vi "Get Package ID.vi"(0 "SystemLink repo in":T1, 7 "package name":string, 9 "package version":string, 11 "error in (no error)":errorcluster) -> (4 "SystemLink repo out":T1, 8 "package ID":string, 15 "error out":errorcluster)   [LabVIEW 2017, in "SystemLink_Repo_API.lvlib"]
doc: "Returns the Package ID for the specified Package Name and Package Version.\n\nError Handling:\nReturns an error if the specified package and version does not exist in the SystemLink repository."
uses:
  SystemLink_Repo_API.lvlib
  systemlink repo.ctl
  <vilib>/httpClient/ClientHandle.ctl
  <vilib>/httpClient/LabVIEWHTTPClient.lvlib
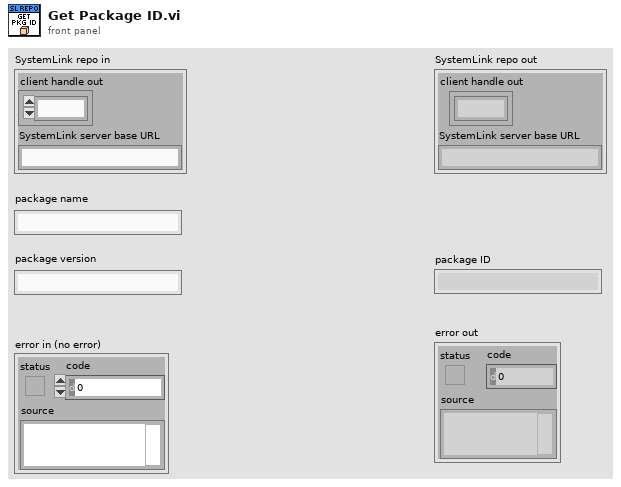
[diagram p1: front panel]
types:
  T1 = typedef "SystemLink_Repo_API.lvlib/systemlink repo.ctl" = cluster{"client handle out":T2, "SystemLink server base URL":string}
  T2 = typedef "LabVIEWHTTPClient.lvlib/ClientHandle.ctl" = refnum<k1>
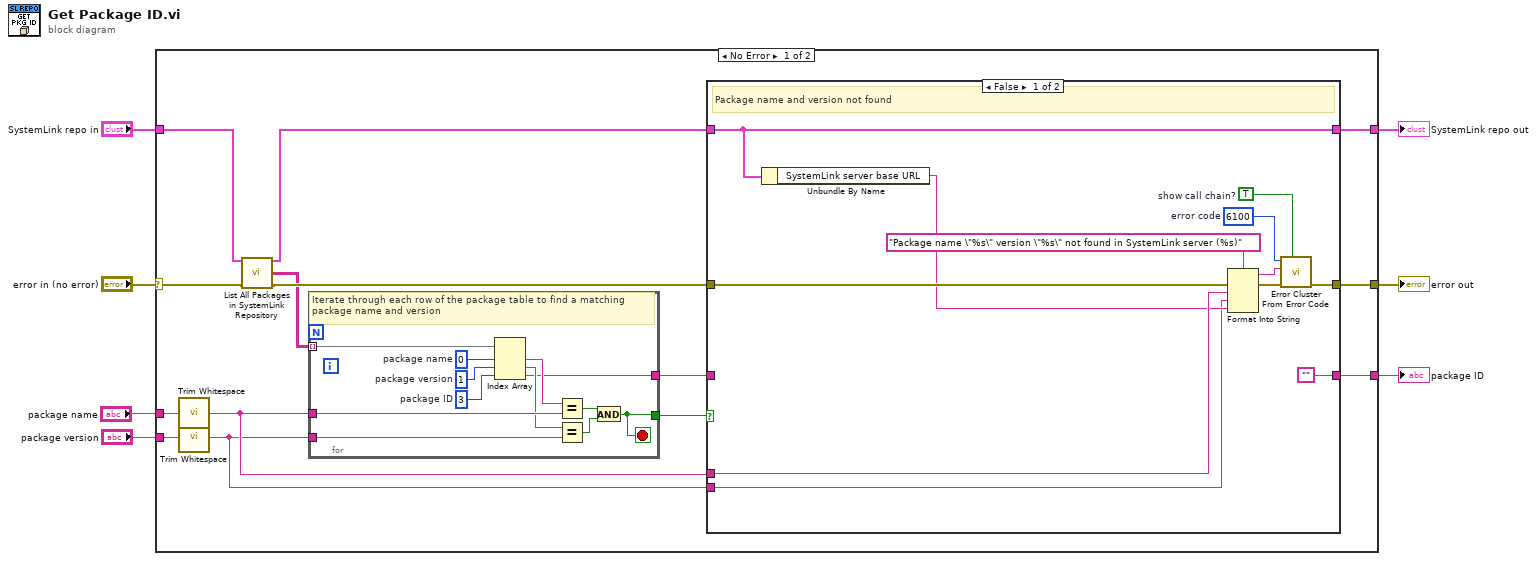
[diagram p0: block diagram]
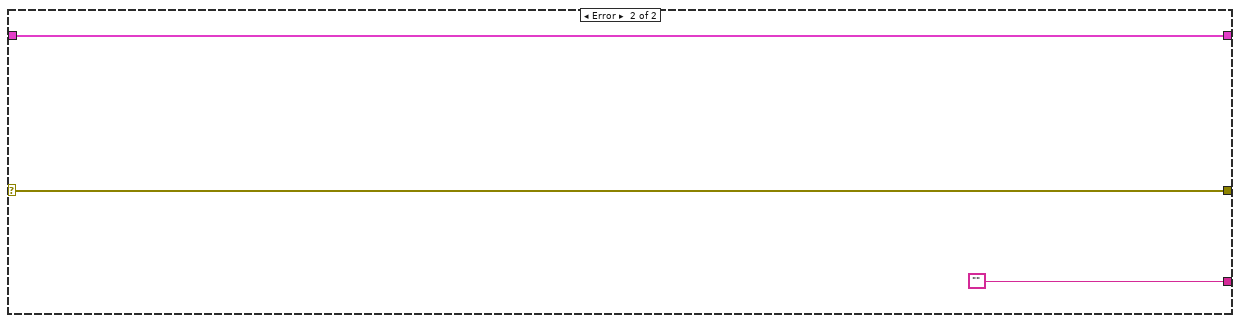
[diagram p3: hidden frame]
diagram:
  n1 = case shown="No Error" "error in (no error)" {
    selector: "error in (no error)" -> [w17 w51]
    tunnel: "SystemLink repo in" -> [w19 w50]
    tunnel: [w21 w51] -> w5
    tunnel: [w20 w50] -> w4
    tunnel: "package name" -> [w15 _]
    tunnel: "package version" -> [w13 _]
    tunnel: [w11 "" ("headers")] -> w1
    frame No Error {
      n2 = call <vilib>:"Trim Whitespace.vi"("string"=w15) -> ("trimmed string"=w10:string)  [unwired: 1 in]
      n3 = call <vilib>:"Trim Whitespace.vi"("string"=w13) -> ("trimmed string"=w9:string)  [unwired: 1 in]
      n4 = call "List All Packages in SystemLink Repository.vi"("SystemLink repo in"=w19, "error in (no error)"=w17) -> ("SystemLink repo out"=w18:T1, "packages"=w8:string[][], "error out"=w16:errorcluster)  [unwired: 11 in]
      n5 = for {
        tunnel: w8 -> [w33] mode=indexing
        tunnel: w10 -> [w31]
        tunnel: w9 -> [w29]
        tunnel: [w26] -> w14
        tunnel: [w22] -> w12
        stop <- w26 stop-if-true
        w23 = 3  # package ID
        w24 = 1  # package version
        w25 = 0  # package name
        # "Iterate through each row of the package table to find a matching package name and version"
        n6 = Index Array(array=w33, index #1=w25, index #2=w24, index #3=w23) -> (element #1=w32:string, element #2=w30:string, element #3=w22:string)
        n7 = Equal?(x=w32, y=w31) -> (x = y?=w28:bool)
        n8 = Equal?(x=w30, y=w29) -> (x = y?=w27:bool)
        n9 = And(x=w28, y=w27) -> (x .and. y?=w26:bool)
      }
      n10 = case shown="False" w14 {
        tunnel: w16 -> [w45 w47]
        tunnel: [w44 w47] -> w21
        tunnel: w18 -> [w41 w48]
        tunnel: [w41 w48] -> w20
        tunnel: w10 -> [w40 _]
        tunnel: w9 -> [w35 _]
        tunnel: w12 -> [_ w46]
        tunnel: ["" w46] -> w11
        frame False {
          w37 = TRUE  # show call chain?
          w38 = 6100  # error code
          # "Package name and version not found"
          n11 = Unbundle By Name(w41) -> ("SystemLink server base URL"=w36:string)
          n12 = Format Into String(format string="Package name \"%s\" version \"%s\" not found in SystemLink server (%s)", error in=w45, w40, w35, w36) -> (resulting string=w39:string, error out=w43:errorcluster)  [unwired: 1 in]
          n13 = call <vilib>:"Error Cluster From Error Code.vi"("show call chain? (False)"=w37, "error in (no error)"=w43, "error message (\"\")"=w39, "error code (0)"=w38) -> ("error out"=w44:errorcluster)  [unwired: 5 in]
        }
        frame True {
          # "Package name and version found"
        }
      }
    }
    frame Error {
    }
  }
  "error out" <- w5
  "SystemLink repo out" <- w4
  "package ID" <- w1
